vi "6221 Write.vi"(0 "Arbitrary Waveform\nArray of Channels":T1(array[cluster])=[[{"AC Frequency (kHz)"=0.0, " Initial AC Ampl. (p-p/2)"=0.0, "Final AC Ampl."=0.0, "Initial DC Value"=7.0, "Final DC Value"=1.0, "Constant/Tau"=2.0, "Gamma AC"=1.0, "String"="Channel 0 A", "Gamma DC/Beta"=1.0}, {"AC Frequency (kHz)"=40.0, " Initial AC Ampl. (p-p/2)"=0.0, "Final AC Ampl."=0.0, "Initial DC Value"=1.0, "Final DC Value"=1.0, "Constant/Tau"=2.0, "Gamma AC"=1.0, "String"="Channel 0 B", "Gamma DC/Beta"=1.0}, {"AC Frequency (kHz)"=40.0, " Initial AC Ampl. (p-p/2)"=0.0, "Final AC Ampl."=0.0, "Initial DC Value"=1.0, "Final DC Value"=1.0, "Constant/Tau"=2.0, "Gamma AC"=1.0, "String"="Channel 0 C", "Gamma DC/Beta"=1.0}, {"AC Frequency (kHz)"=0.0, " Initial AC Ampl. (p-p/2)"=0.0, "Final AC Ampl."=0.0, "Initial DC Value"=1.0, "Final DC Value"=7.0, "Constant/Tau"=2.0, "Gamma AC"=0.0, "String"="Channel 0 D", "Gamma DC/Beta"=1.0}, {"AC Frequency (kHz)"=0.0, " Initial AC Ampl. (p-p/2)"=0.0, "Final AC Ampl."=0.0, "Initial DC Value"=7.0, "Final DC Value"=6.0, "Constant/Tau"=2.0, "Gamma AC"=0.0, "String"="Channel 0 E", "Gamma DC/Beta"=1.0}], [{"AC Frequency (kHz)"=10.0, " Initial AC Ampl. (p-p/2)"=5.0, "Final AC Ampl."=0.0, "Initial DC Value"=0.2, "Final DC Value"=0.16, "Constant/Tau"=0.25, "Gamma AC"=1.0, "String"="Channel 1 A", "Gamma DC/Beta"=1.0}, {"AC Frequency (kHz)"=10.0, " Initial AC Ampl. (p-p/2)"=5.0, "Final AC Ampl."=0.0, "Initial DC Value"=0.16, "Final DC Value"=0.16, "Constant/Tau"=0.25, "Gamma AC"=1.0, "String"="Channel 1 B", "Gamma DC/Beta"=1.0}, {"AC Frequency (kHz)"=10.0, " Initial AC Ampl. (p-p/2)"=0.0, "Final AC Ampl."=0.0, "Initial DC Value"=0.0, "Final DC Value"=0.0, "Constant/Tau"=0.25, "Gamma AC"=1.0, "String"="Channel 1 C", "Gamma DC/Beta"=1.0}, {"AC Frequency (kHz)"=0.0, " Initial AC Ampl. (p-p/2)"=0.0, "Final AC Ampl."=0.0, "Initial DC Value"=1.0, "Final DC Value"=1.0, "Constant/Tau"=199.2, "Gamma AC"=0.0, "String"="Channel 1 D", "Gamma DC/Beta"=1.0}, {"AC Frequency (kHz)"=0.0, " Initial AC Ampl. (p-p/2)"=0.0, "Final AC Ampl."=0.0, "Initial DC Value"=1.0, "Final DC Value"=1.0, "Constant/Tau"=199.2, "Gamma AC"=0.0, "String"="Channel 1 E", "Gamma DC/Beta"=1.0}], [{"AC Frequency (kHz)"=10.0, " Initial AC Ampl. (p-p/2)"=0.0, "Final AC Ampl."=0.0, "Initial DC Value"=0.007, "Final DC Value"=0.06, "Constant/Tau"=0.0, "Gamma AC"=1.0, "String"="Channel 2 A", "Gamma DC/Beta"=1.0}, {"AC Frequency (kHz)"=10.0, " Initial AC Ampl. (p-p/2)"=0.0, "Final AC Ampl."=0.0, "Initial DC Value"=0.06, "Final DC Value"=0.06, "Constant/Tau"=0.0, "Gamma AC"=1.0, "String"="Channel 2 B", "Gamma DC/Beta"=1.0}, {"AC Frequency (kHz)"=10.0, " Initial AC Ampl. (p-p/2)"=0.0, "Final AC Ampl."=0.0, "Initial DC Value"=0.0, "Final DC Value"=0.0, "Constant/Tau"=0.0, "Gamma AC"=1.0, "String"="Channel 2 C", "Gamma DC/Beta"=1.0}, {"AC Frequency (kHz)"=0.0, " Initial AC Ampl. (p-p/2)"=0.0, "Final AC Ampl."=0.0, "Initial DC Value"=1.0, "Final DC Value"=1.0, "Constant/Tau"=199.2, "Gamma AC"=0.0, "String"="", "Gamma DC/Beta"=1.0}, {"AC Frequency (kHz)"=0.0, " Initial AC Ampl. (p-p/2)"=0.0, "Final AC Ampl."=0.0, "Initial DC Value"=1.0, "Final DC Value"=1.0, "Constant/Tau"=199.2, "Gamma AC"=0.0, "String"="", "Gamma DC/Beta"=1.0}], [{"AC Frequency (kHz)"=10.0, " Initial AC Ampl. (p-p/2)"=0.0, "Final AC Ampl."=0.0, "Initial DC Value"=1.0, "Final DC Value"=1.0, "Constant/Tau"=199.2, "Gamma AC"=1.0, "String"="Channel 3 A", "Gamma DC/Beta"=1.0}, {"AC Frequency (kHz)"=10.0, " Initial AC Ampl. (p-p/2)"=0.0, "Final AC Ampl."=0.0, "Initial DC Value"=1.0, "Final DC Value"=1.0, "Constant/Tau"=199.2, "Gamma AC"=1.0, "String"="Channel 3 B", "Gamma DC/Beta"=1.0}, {"AC Frequency (kHz)"=10.0, " Initial AC Ampl. (p-p/2)"=0.0, "Final AC Ampl."=0.0, "Initial DC Value"=1.0, "Final DC Value"=1.0, "Constant/Tau"=199.2, "Gamma AC"=1.0, "String"="Channel 3 C", "Gamma DC/Beta"=1.0}, {"AC Frequency (kHz)"=0.0, " Initial AC Ampl. (p-p/2)"=0.0, "Final AC Ampl."=0.0, "Initial DC Value"=1.0, "Final DC Value"=1.0, "Constant/Tau"=199.2, "Gamma AC"=0.0, "String"="", "Gamma DC/Beta"=1.0}, {"AC Frequency (kHz)"=0.0, " Initial AC Ampl. (p-p/2)"=0.0, "Final AC Ampl."=0.0, "Initial DC Value"=1.0, "Final DC Value"=1.0, "Constant/Tau"=199.2, "Gamma AC"=0.0, "String"="", "Gamma DC/Beta"=1.0}], [{"AC Frequency (kHz)"=10.0, " Initial AC Ampl. (p-p/2)"=0.0, "Final AC Ampl."=0.0, "Initial DC Value"=-0.1, "Final DC Value"=-0.04, "Constant/Tau"=199.2, "Gamma AC"=1.0, "String"="Channel 4 A", "Gamma DC/Beta"=1.0}, {"AC Frequency (kHz)"=10.0, " Initial AC Ampl. (p-p/2)"=0.0, "Final AC Ampl."=0.0, "Initial DC Value"=-0.1, "Final DC Value"=-0.04, "Constant/Tau"=199.2, "Gamma AC"=1.0, "String"="Channel 4 B", "Gamma DC/Beta"=1.0}, {"AC Frequency (kHz)"=10.0, " Initial AC Ampl. (p-p/2)"=0.0, "Final AC Ampl."=0.0, "Initial DC Value"=-0.1, "Final DC Value"=-0.04, "Constant/Tau"=199.2, "Gamma AC"=1.0, "String"="Channel 4 C", "Gamma DC/Beta"=1.0}, {"AC Frequency (kHz)"=0.0, " Initial AC Ampl. (p-p/2)"=0.0, "Final AC Ampl."=0.0, "Initial DC Value"=1.0, "Final DC Value"=1.0, "Constant/Tau"=199.2, "Gamma AC"=0.0, "String"="", "Gamma DC/Beta"=1.0}, {"AC Frequency (kHz)"=0.0, " Initial AC Ampl. (p-p/2)"=0.0, "Final AC Ampl."=0.0, "Initial DC Value"=1.0, "Final DC Value"=1.0, "Constant/Tau"=199.2, "Gamma AC"=0.0, "String"="", "Gamma DC/Beta"=1.0}], [{"AC Frequency (kHz)"=10.0, " Initial AC Ampl. (p-p/2)"=0.0, "Final AC Ampl."=0.0, "Initial DC Value"=-0.1, "Final DC Value"=-0.04, "Constant/Tau"=199.2, "Gamma AC"=1.0, "String"="Channel 5 A", "Gamma DC/Beta"=1.0}, {"AC Frequency (kHz)"=10.0, " Initial AC Ampl. (p-p/2)"=0.0, "Final AC Ampl."=0.0, "Initial DC Value"=-0.1, "Final DC Value"=-0.04, "Constant/Tau"=199.2, "Gamma AC"=1.0, "String"="Channel 5 B", "Gamma DC/Beta"=1.0}, {"AC Frequency (kHz)"=10.0, " Initial AC Ampl. (p-p/2)"=0.0, "Final AC Ampl."=0.0, "Initial DC Value"=-0.1, "Final DC Value"=-0.04, "Constant/Tau"=199.2, "Gamma AC"=1.0, "String"="Channel 5 C", "Gamma DC/Beta"=1.0}, {"AC Frequency (kHz)"=0.0, " Initial AC Ampl. (p-p/2)"=0.0, "Final AC Ampl."=0.0, "Initial DC Value"=1.0, "Final DC Value"=1.0, "Constant/Tau"=199.2, "Gamma AC"=0.0, "String"="", "Gamma DC/Beta"=1.0}, {"AC Frequency (kHz)"=0.0, " Initial AC Ampl. (p-p/2)"=0.0, "Final AC Ampl."=0.0, "Initial DC Value"=1.0, "Final DC Value"=1.0, "Constant/Tau"=199.2, "Gamma AC"=0.0, "String"="", "Gamma DC/Beta"=1.0}], [{"AC Frequency (kHz)"=10.0, " Initial AC Ampl. (p-p/2)"=0.0, "Final AC Ampl."=0.0, "Initial DC Value"=-0.1, "Final DC Value"=-0.04, "Constant/Tau"=199.2, "Gamma AC"=1.0, "String"="Channel 6 A", "Gamma DC/Beta"=1.0}, {"AC Frequency (kHz)"=10.0, " Initial AC Ampl. (p-p/2)"=0.0, "Final AC Ampl."=0.0, "Initial DC Value"=-0.1, "Final DC Value"=-0.04, "Constant/Tau"=199.2, "Gamma AC"=1.0, "String"="Channel 6 B", "Gamma DC/Beta"=1.0}, {"AC Frequency (kHz)"=10.0, " Initial AC Ampl. (p-p/2)"=0.0, "Final AC Ampl."=0.0, "Initial DC Value"=-0.1, "Final DC Value"=-0.04, "Constant/Tau"=199.2, "Gamma AC"=1.0, "String"="Channel 6 C", "Gamma DC/Beta"=1.0}, {"AC Frequency (kHz)"=0.0, " Initial AC Ampl. (p-p/2)"=0.0, "Final AC Ampl."=0.0, "Initial DC Value"=1.0, "Final DC Value"=1.0, "Constant/Tau"=199.2, "Gamma AC"=0.0, "String"="", "Gamma DC/Beta"=1.0}, {"AC Frequency (kHz)"=0.0, " Initial AC Ampl. (p-p/2)"=0.0, "Final AC Ampl."=0.0, "Initial DC Value"=1.0, "Final DC Value"=1.0, "Constant/Tau"=199.2, "Gamma AC"=0.0, "String"="", "Gamma DC/Beta"=1.0}], [{"AC Frequency (kHz)"=10.0, " Initial AC Ampl. (p-p/2)"=0.0, "Final AC Ampl."=0.0, "Initial DC Value"=-0.1, "Final DC Value"=-0.04, "Constant/Tau"=199.2, "Gamma AC"=1.0, "String"="Channel 7 A", "Gamma DC/Beta"=1.0}, {"AC Frequency (kHz)"=10.0, " Initial AC Ampl. (p-p/2)"=0.0, "Final AC Ampl."=0.0, "Initial DC Value"=-0.1, "Final DC Value"=-0.04, "Constant/Tau"=199.2, "Gamma AC"=1.0, "String"="Channel 7 B", "Gamma DC/Beta"=1.0}, {"AC Frequency (kHz)"=10.0, " Initial AC Ampl. (p-p/2)"=0.0, "Final AC Ampl."=0.0, "Initial DC Value"=-0.1, "Final DC Value"=-0.04, "Constant/Tau"=199.2, "Gamma AC"=1.0, "String"="Channel 7 C", "Gamma DC/Beta"=1.0}, {"AC Frequency (kHz)"=0.0, " Initial AC Ampl. (p-p/2)"=0.0, "Final AC Ampl."=0.0, "Initial DC Value"=1.0, "Final DC Value"=1.0, "Constant/Tau"=199.2, "Gamma AC"=0.0, "String"="", "Gamma DC/Beta"=1.0}, {"AC Frequency (kHz)"=0.0, " Initial AC Ampl. (p-p/2)"=0.0, "Final AC Ampl."=0.0, "Initial DC Value"=1.0, "Final DC Value"=1.0, "Constant/Tau"=199.2, "Gamma AC"=0.0, "String"="", "Gamma DC/Beta"=1.0}]] {"Gamma DC/Beta" format="%.2f"; "Gamma AC" format="%.2f"; "Constant/Tau" min=0.0 max=240.0 format="%.4f"; "Final DC Value" format="%.3f"; "Initial DC Value" format="%.3f"; "Final AC Ampl." format="%.3f"; "Initial AC Ampl. (p-p/2)" format="%.3f"; "AC Frequency (kHz)" format="%.2f"}, 2 "Channel to plot":i32 min=0 max=7, 3 "Unit Conversions":u16[](array[ring])=[0, 0, 2, 3, 4, 0, 0, 0] items=["Volts-to-Volts Power Law", "Evaporation Formula", "Dimple Evaporation"], 4 "Interval Lengths (ms)":dbl[](array[numeric])=[120.0, 16.0, 484.0, 700.0, 100.0] format="%.3f", 5 "Channel Controls":bool[](array[boolean])=[TRUE, TRUE, FALSE, FALSE, FALSE, FALSE, FALSE, FALSE], 6 "ON or OFF?":bool[](array[boolean])=[TRUE, TRUE, TRUE, FALSE, FALSE], 11 "error in":errorcluster, 12 "Dither Control":u16(ring)=1 items=["Disable Dither", "Enable Dither"]) -> (9 "Sampling Rate":dbl=2882.3529411764707 format="%.2f", 10 "= Total Waveform\nTime (ms)":dbl=1420.0 format="%.3f", 13 "Waveform on Channel to Plot":cluster{dbl[], dbl[]}(graph), 14 "signal out":waveform(dbl)[](graph)=[{"t0"=timestamp(0 s since 1904-01-01), "dt"=0.00034693877551020405, "Y"=array[4091 elements]}, {"t0"=timestamp(0 s since 1904-01-01), "dt"=0.00034693877551020405, "Y"=array[4091 elements]}], 15 "error out":errorcluster)   [LabVIEW 2013]
uses:
  <vilib>/Utility/error.llb/DialogType.ctl
  <vilib>/DAQmx/write.llb/DAQmx Write (Analog 1D Wfm NChan NSamp).vi
  <vilib>/DAQmx/configure/timing.llb/DAQmx Timing (Sample Clock).vi
  <vilib>/DAQmx/create/channels.llb/DAQmx Create Channel (CO-Pulse Generation-Frequency).vi
  <vilib>/DAQmx/configure/timing.llb/DAQmx Timing (Implicit).vi
  <vilib>/DAQmx/configure/trigger.llb/DAQmx Start Trigger (Digital Edge).vi
  <vilib>/DAQmx/miscellaneous.llb/DAQmx Fill In Error Info.vi
  <resource>/objmgr/daqmx.rc
panel:
  in  "Case Constant\n(See Context Help) 3":bool=TRUE
  in  "Case Constant\n(See Context Help) 2":bool
  in  "Dither Control":u16
  in  "Case Constant\n(See Context Help)":bool
  in  "Dither Control":u16
  out "Pmod Graph":dbl[][](graph)
  out "wvfrm size":i32=4091
  out "x+y 2":dbl=1.42
  out "Numeric":i32=287
  out "6221 counter task out":refnum<k21>="Counter Output"
  out "6221 adiabatic loading task out":refnum<k21>="Adiabatic Loading"
  out "Array":dbl[][](array[numeric])
  out "6221 Status":string="PCI-6221 OK"
  out "total points":dbl=4092.0 format="%.2f"
  out "Points per Segment":dbl[](array[numeric])=[345.0, 46.0, 1395.0, 2017.0, 288.0] format="%.2f"
  # "Warning! Constant for interval A does not set all intervals for 86 Sr frequency"
  # "Controls"
  # "Volts to Volts Power Law Formula\nf100=DCinitial +(DCfinal-DCinitial)*(time/intervaltime)**gammaDC;"
  # "Don't change"
  # "Note: B-field to Voltage\nConversion not yet\nimplemented.  Must \ninsert appropriate\nformulae."
  # "CH 0"
  # "CH 1"
  # "Evaporation Formula\nf100=Initial/((1+(time/tau))**beta)+Final;"
  # "Initial DC = U1, Constant = Tau\nGamma DC = Beta"
  # "Interval A"
  # "Interval B"
  # "Interval C"
  # "Interval D"
  # "Interval E"
  # "Interval F"
  # "Output"
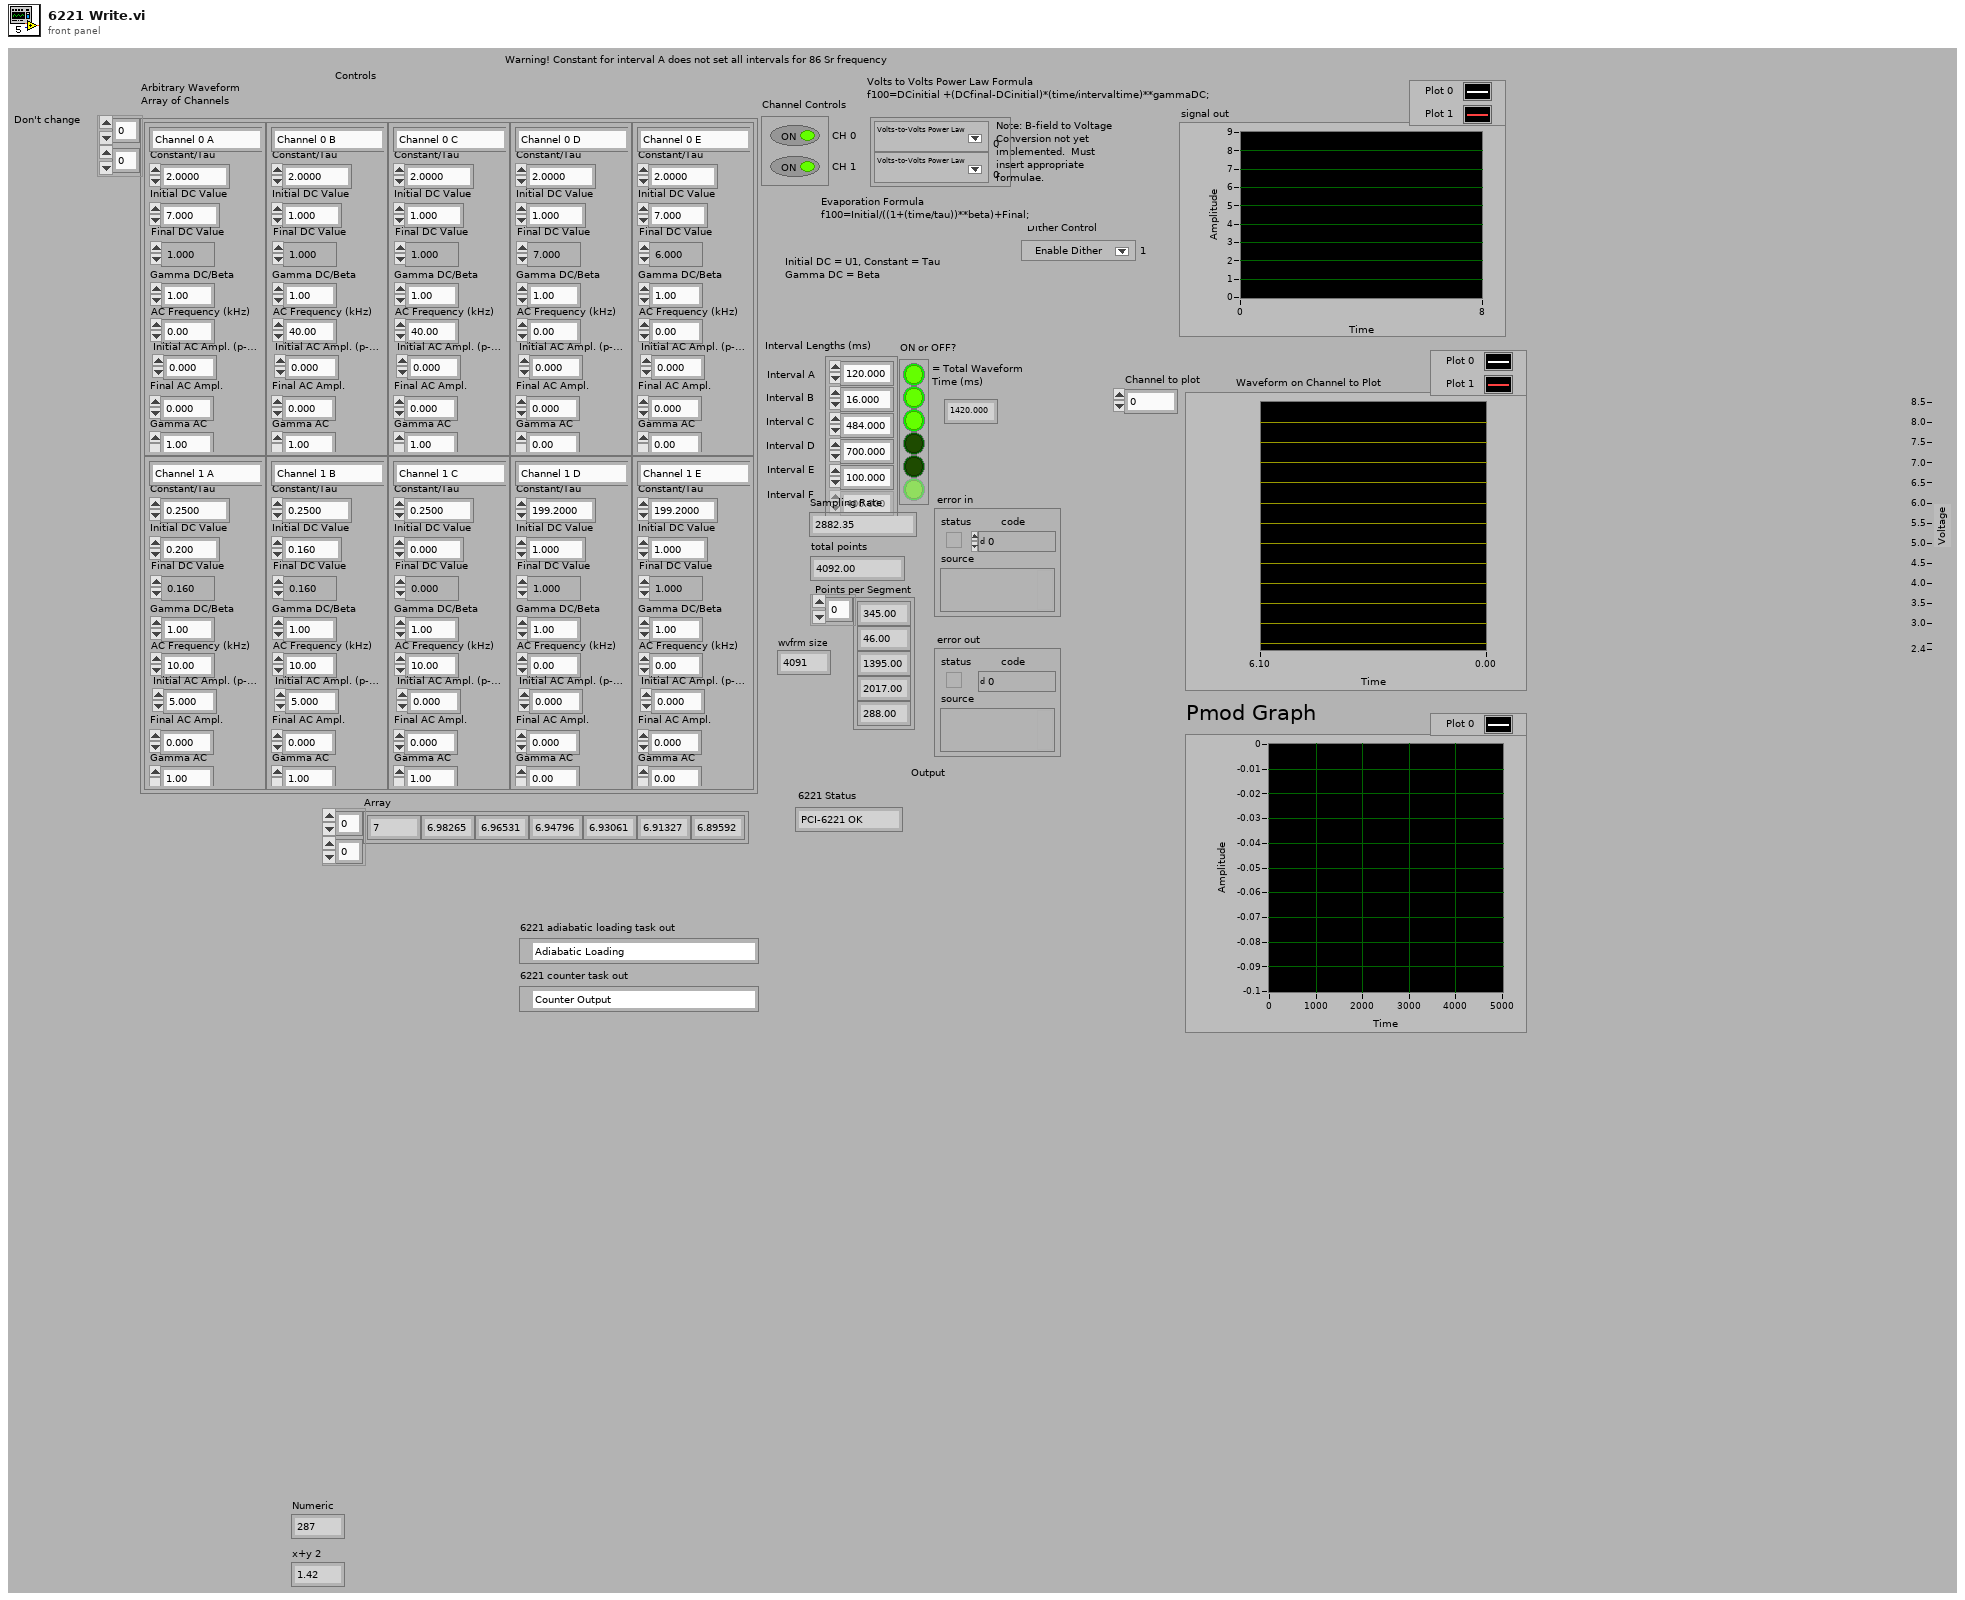
[diagram p1: front panel]
types:
  T1 = cluster{"AC Frequency (kHz)":dbl, " Initial AC Ampl. (p-p/2)":dbl, "Final AC Ampl.":dbl, "Initial DC Value":dbl, "Final DC Value":dbl, "Constant/Tau":dbl, "Gamma AC":dbl, "String":string, "Gamma DC/Beta":dbl}[][]
  T2 = cluster{"AC Frequency (kHz)":dbl, " Initial AC Ampl. (p-p/2)":dbl, "Final AC Ampl.":dbl, "Initial DC Value":dbl, "Final DC Value":dbl, "Constant/Tau":dbl, "Gamma AC":dbl, "String":string, "Gamma DC/Beta":dbl}
  T3 = typedef "DialogType.ctl" = u16
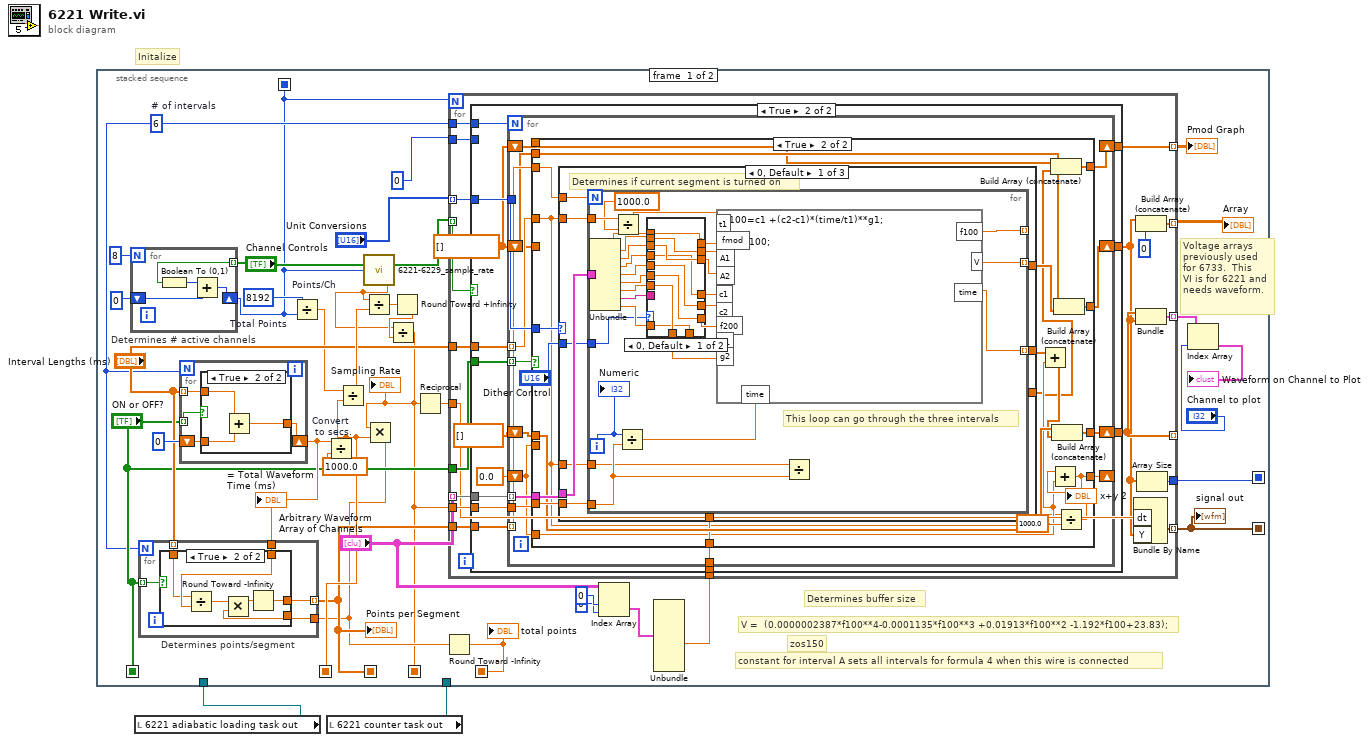
[diagram p0: block diagram]
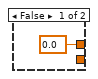
[diagram p2: hidden frame]
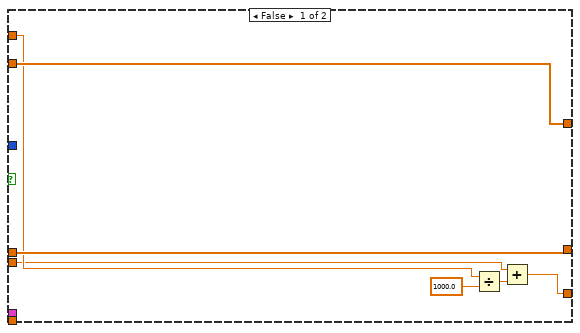
[diagram p5: hidden frame]
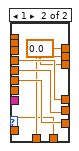
[diagram p6: hidden frame]
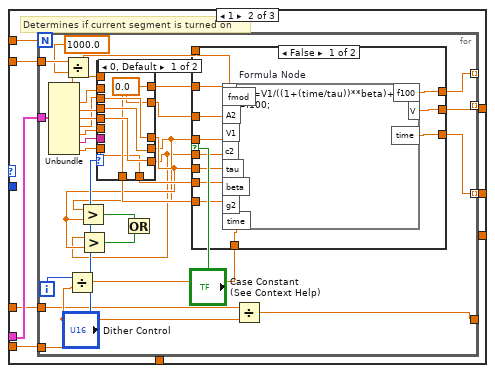
[diagram p7: hidden frame]
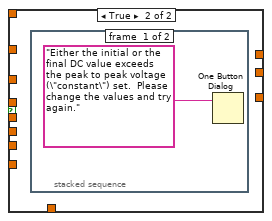
[diagram p8: hidden frame]
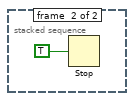
[diagram p9: hidden frame]
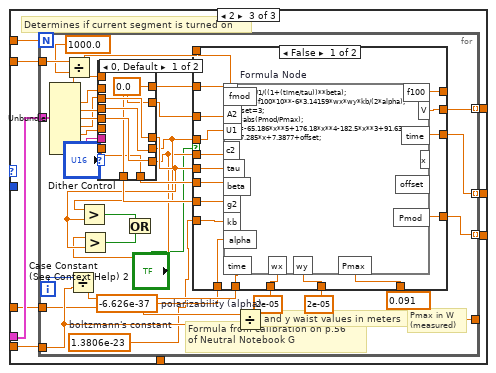
[diagram p11: hidden frame]
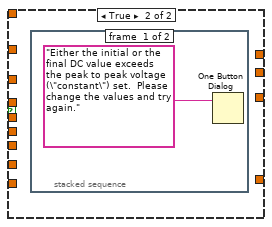
[diagram p12: hidden frame]
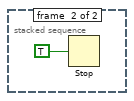
[diagram p13: hidden frame]
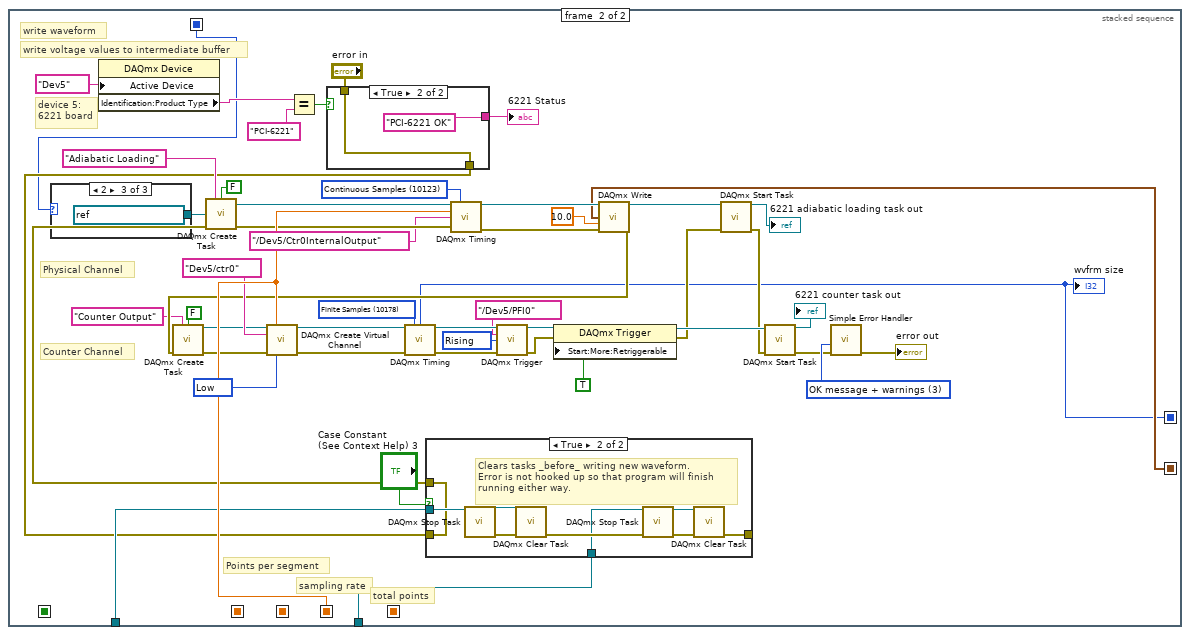
[diagram p15: hidden frame]
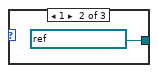
[diagram p17: hidden frame]
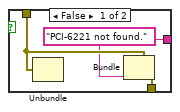
[diagram p19: hidden frame]
diagram:
  # "Initalize"
  n1 = local read "6221 adiabatic loading task out"() -> (w2:refnum<k21>)
  n2 = local read "6221 counter task out"() -> (w1:refnum<k21>)
  n3 = stacked-sequence {
    seq-local: [w10 _] -> [_ w356]
    seq-local: [w22 _] -> [_ _]
    seq-local: ["ON or OFF?" _] -> [_ _]
    seq-local: [w19 _] -> [_ _]
    seq-local: [w24 _] -> [_ _]
    seq-local: [w8 _] -> [_ w330]
    seq-local: [w3 _] -> [_ w331]
    seq-local: [w7 _] -> [_ w329]
    tunnel: w2 -> [_ w341]
    tunnel: w1 -> [_ w342]
    frame #0 {
      w6 = 6  # # of intervals
      w38 = 8192  # Total Points
      # "Voltage arrays\npreviously used\nfor 6733.  This\nVI is for 6221 and\nneeds waveform."
      # "zos150"
      # "Determines buffer size"
      # "constant for interval A sets all intervals for formula 4 when this wire is connected"
      # "V =  (0.0000002387*f100**4-0.0001135*f100**3 +0.01913*f100**2 -1.192*f100+23.83);"
      n4 = for "Determines # active channels" {
        N: 8 -> [_]
        tunnel: "Channel Controls" -> [w62] mode=indexing
        shift-right: [w59] -> w3
        shift-left: 0 -> [w60]
        n5 = Boolean To (0,1)(Boolean=w62) -> (0, 1=w61:i16)
        n6 = Add(x=w61, y=w60) -> (x+y=w59:i32)
      }
      n7 = for {
        N: w6 -> [_]
        tunnel: "Interval Lengths (ms)" -> [w52] mode=indexing
        tunnel: "ON or OFF?" -> [w54] mode=indexing
        shift-right: [w51] -> w25
        shift-left: 0 -> [w53]
        n8 = case shown="True" w54 {
          tunnel: w53 -> [w55 w58]
          tunnel: w52 -> [_ w57]
          tunnel: [w55 w56] -> w51
          frame False {
          }
          frame True {
            n9 = Add(x=w57, y=w58) -> (x+y=w56:dbl)
          }
        }
      }
      "= Total Waveform\nTime (ms)" <- w25
      n10 = Divide "Points/Ch"(x=w38, y=w3) -> (x/y=w23:dbl)
      n11 = Divide "Convert\n to secs."(x=w25, y=1000.0) -> (x/y=w24:dbl)
      n12 = Divide(x=w23, y=w24) -> (x/y=w30:dbl)
      n13 = call "6221-6229_sample_rate.vi"("# of output channels"=w3) -> ("Sampling rate"=w4:dbl)
      n14 = Divide(x=w4, y=w30) -> (x/y=w29:dbl)
      n15 = Round Toward +Infinity(x=w29) -> (ceil(x): smallest int >= x=w28:dbl)
      n16 = Divide(x=w4, y=w28) -> (x/y=w10:dbl)
      "Sampling Rate" <- w10
      n17 = Multiply(x=w10, y=w24) -> (x*y=w20:dbl)
      n18 = for "Determines points/segment" {
        N: w6 -> [_]
        tunnel: "ON or OFF?" -> [w43] mode=indexing
        tunnel: "Interval Lengths (ms)" -> [w42] mode=indexing
        tunnel: w25 -> [w41]
        tunnel: [w40] -> w22 mode=indexing
        tunnel: w20 -> [w39]
        n19 = case shown="True" w43 {
          tunnel: w42 -> [_ w49]
          tunnel: w41 -> [_ w50]
          tunnel: [0.0 w46] -> w40
          tunnel: w39 -> [_ w47]
          frame False {
          }
          frame True {
            n20 = Divide(x=w49, y=w50) -> (x/y=w48:dbl)
            n21 = Multiply(x=w48, y=w47) -> (x*y=w45:dbl)
            n22 = Round Toward -Infinity(1:w45) -> (0:w46:dbl)
          }
        }
      }
      "Points per Segment" <- w22
      n23 = Reciprocal(x=w10) -> (1/x=w9:dbl)
      n24 = Round Toward -Infinity(1:w20) -> (0:w19:dbl)
      "total points" <- w19
      n25 = Index Array(array="Arbitrary Waveform\nArray of Channels", index (row)=0, index (col)=0 ("disabled index (col)")) -> (element=w14:T2)
      n26 = Unbundle(w14) -> ("Constant/Tau"=w13:dbl)  [unwired: 8 out]
      n27 = for {
        N: w3 -> [_]
        tunnel: "Channel Controls" -> [w81] mode=indexing
        tunnel: 0 -> [w80]
        tunnel: "Unit Conversions" -> [w78] mode=indexing
        tunnel: "Arbitrary Waveform\nArray of Channels" -> [w79] mode=indexing
        tunnel: w22 -> [w77]
        tunnel: w10 -> [w76]
        tunnel: "Interval Lengths (ms)" -> [w75]
        tunnel: "ON or OFF?" -> [w74]
        tunnel: [w67] -> _ mode=indexing
        tunnel: [w71] -> w18 mode=indexing
        tunnel: [w73] -> w26 mode=indexing
        tunnel: w13 -> [w70]
        tunnel: w9 -> [w69]
        tunnel: [w68] -> w8 mode=indexing
        tunnel: [w65] -> w7
        tunnel: w6 -> [w64]
        tunnel: [w63] -> w5 mode=indexing
        n28 = case shown="True" w81 {
          tunnel: w80 -> [_ _]
          tunnel: w79 -> [_ w95]
          tunnel: w78 -> [_ w94]
          tunnel: w77 -> [_ w93]
          tunnel: w76 -> [_ w92]
          tunnel: w75 -> [_ w91]
          tunnel: w74 -> [_ w90]
          tunnel: [_ w89] -> w66
          tunnel: w70 -> [_ w88]
          tunnel: [_ w86] -> w67
          tunnel: w64 -> [_ w84]
          tunnel: [_ w82] -> w63
          frame False {
          }
          frame True {
            w83 = dbl[] []
            n29 = for {
              N: w84 -> [_]
              tunnel: w95 -> [w108] mode=indexing
              tunnel: w94 -> [w110]
              tunnel: w93 -> [w109] mode=indexing
              tunnel: w92 -> [w107]
              tunnel: w91 -> [w106] mode=indexing
              tunnel: w90 -> [w105] mode=indexing
              shift-right: [w99] -> w86
              shift-left: dbl[] [] -> [w104]
              shift-right: [w103] -> _
              shift-left: 0.0 -> [w98]
              shift-right: [w102] -> w89
              shift-left: w83 -> [w101]
              tunnel: w88 -> [w100]
              shift-right: [w96] -> w82
              shift-left: w83 -> [w97]
              n30 = case shown="True" w105 {
                tunnel: w110 -> [_ w131]
                tunnel: w109 -> [_ w127]
                tunnel: w108 -> [_ w138]
                tunnel: w107 -> [_ w137]
                tunnel: w106 -> [w113 w121]
                tunnel: [w117 w136] -> w99
                tunnel: w104 -> [w117 w135]
                tunnel: [w112 w128] -> w103
                tunnel: [w116 w134] -> w102
                tunnel: w101 -> [_ w132]
                tunnel: w101 -> [w116 _]
                tunnel: w100 -> [_ w129]
                tunnel: w98 -> [_ w122]
                tunnel: w98 -> [w111 _]
                tunnel: [_ w119] -> w96
                tunnel: w97 -> [_ w118]
                frame False {
                  n31 = Divide(x=w113, y=1000.0) -> (x/y=w115:dbl)
                  n32 = Add(x=w111, y=w115) -> (x+y=w112:dbl)
                }
                frame True {
                  n33 = case shown="0, Default" w131 {
                    tunnel: w127 -> [w146 w195 w260]
                    tunnel: w138 -> [w145 w194 w259]
                    tunnel: w137 -> [w141 w190 w255]
                    tunnel: w121 -> [w144 w193 w258]
                    tunnel: [w143 w192 w257] -> w133
                    tunnel: [w142 w191 w256] -> w124
                    tunnel: w121 -> [w140 w189 w254]
                    tunnel: "Dither Control" -> [w139 _ _]
                    tunnel: w129 -> [_ _ _]
                    tunnel: [_ _ w253] -> w120
                    frame 0, Default {
                      # "Determines if current segment is turned on"
                      n34 = for {
                        N: w146 -> [_]
                        tunnel: w145 -> [w175]
                        tunnel: w141 -> [w154]
                        tunnel: w144 -> [w174]
                        tunnel: [w152] -> w143 mode=indexing
                        tunnel: [w153] -> w142 mode=indexing
                        tunnel: [w151] -> _ mode=indexing
                        tunnel: w140 -> [w149]
                        tunnel: w139 -> [w150]
                        i -> [w172]
                        # "Volts-to-Volts Power Law"
                        # "This loop can go through the three intervals"
                        n35 = Unbundle(w175) -> ("AC Frequency (kHz)"=w168:dbl, "Initial AC Ampl. (p-p/2)"=w167:dbl, "Final AC Ampl."=w166:dbl, "Initial DC Value"=w147:dbl, "Final DC Value"=w165:dbl, "Constant/Tau"=w169:dbl, "Gamma AC"=w170:dbl, "String"=w171:string, "Gamma DC/Beta"=w156:dbl)
                        n36 = Divide(x=w174, y=1000.0) -> (x/y=w164:dbl)
                        n37 = Divide(x=w172, y=w154) -> (x/y=w148:dbl)
                        n38 = case shown="0, Default" w150 {
                          tunnel: w171 -> [_ _]
                          tunnel: w170 -> [w177 _]
                          tunnel: w169 -> [w178 w186]
                          tunnel: w168 -> [w183 _]
                          tunnel: w167 -> [w182 _]
                          tunnel: w166 -> [w181 _]
                          tunnel: w147 -> [w180 w188]
                          tunnel: w165 -> [w179 w187]
                          tunnel: [w183 w185] -> w163
                          tunnel: [w182 w185] -> w162
                          tunnel: [w181 w185] -> w161
                          tunnel: [w180 w188] -> w160
                          tunnel: [w179 w187] -> w159
                          tunnel: [w178 w186] -> w158
                          tunnel: [w177 w185] -> w157
                          tunnel: w156 -> [w176 w184]
                          tunnel: [w176 w184] -> w155
                          frame 0, Default {
                          }
                          frame 1 {
                            w185 = 0.0 ("AC Frequency (kHz)")
                          }
                        }
                        n39 = formula code="f100=c1 +(c2-c1)*(time/t1)**g1;\n\nV = f100;"("c1"=w160, "time"=w148, "t1"=w164, "c2"=w159, "f200"=w158, "fmod"=w163, "A1"=w162, "A2"=w161, "g1"=w155, "g2"=w157) -> ("f100"=w151:dbl, "time"=w153:dbl, "V"=w152:dbl)
                        n40 = Divide(x=w149, y=w154) -> ()  [unwired: 1 out]
                        "Numeric" <- w172
                      }
                    }
                    frame 1 {
                      # "Determines if current segment is turned on"
                      n41 = for {
                        N: w195 -> [_]
                        tunnel: w194 -> [w226]
                        tunnel: w190 -> [w210]
                        tunnel: w193 -> [w222]
                        tunnel: [w225] -> w192 mode=indexing
                        tunnel: [w224] -> w191 mode=indexing
                        tunnel: [w223] -> _ mode=indexing
                        tunnel: [w209] -> _
                        tunnel: w189 -> [w197]
                        i -> [w220]
                        n42 = Unbundle(w226) -> ("AC Frequency (kHz)"=w203:dbl, "Final AC Ampl."=w204:dbl, "Initial DC Value"=w207:dbl, "Final DC Value"=w206:dbl, "Constant/Tau"=w205:dbl, "Gamma AC"=w218:dbl, "String"=w219:string, "Gamma DC/Beta"=w213:dbl)  [unwired: 1 out]
                        n43 = Divide(x=w222, y=1000.0) -> (x/y=w217:dbl)
                        n44 = Divide(x=w220, y=w210) -> (x/y=w211:dbl)
                        n45 = case shown="0, Default" "Dither Control" {
                          tunnel: w219 -> [_ _]
                          tunnel: w218 -> [_ w248]
                          tunnel: w206 -> [w243 w249]
                          tunnel: w204 -> [_ w252]
                          tunnel: w205 -> [w245 w251]
                          tunnel: w207 -> [w244 w250]
                          tunnel: [w242 w246] -> w216
                          tunnel: [w242 w252] -> w215
                          tunnel: [w245 w251] -> w200
                          tunnel: [w244 w250] -> w199
                          tunnel: [w243 w249] -> w198
                          tunnel: [w242 w248] -> w214
                          tunnel: w213 -> [w241 w247]
                          tunnel: [w241 w247] -> w212
                          tunnel: w203 -> [_ w246]
                          frame 0, Default {
                            w242 = 0.0 ("AC Frequency (kHz)")
                          }
                          frame 1 {
                          }
                        }
                        n46 = Greater?(x=w199, y=w200) -> (0:w201:bool)
                        n47 = Greater?(x=w198, y=w200) -> (0:w202:bool)
                        n48 = Or(x=w201, y=w202) -> ()  [unwired: 1 out]
                        n49 = case shown="False" "Case Constant\n(See Context Help)" {
                          tunnel: [w238 _] -> w225
                          tunnel: [w237 _] -> w224
                          tunnel: [w236 _] -> w223
                          tunnel: w217 -> [w235 _]
                          tunnel: w216 -> [w234 _]
                          tunnel: w215 -> [w233 _]
                          tunnel: w214 -> [w232 _]
                          tunnel: w212 -> [w231 _]
                          tunnel: w211 -> [w230 _]
                          tunnel: w199 -> [w229 _]
                          tunnel: w198 -> [w228 _]
                          tunnel: w200 -> [w227 _]
                          frame False {
                            # "Evaporative Cooling"
                            n50 = formula code="f100=V1/((1+(time/tau))**beta)+c2;\nV=f100;"("V1"=w229, "time"=w230, "t1"=w235, "c2"=w228, "tau"=w227, "fmod"=w234, "A2"=w233, "beta"=w231, "g2"=w232) -> ("f100"=w236:dbl, "time"=w237:dbl, "V"=w238:dbl)
                          }
                          frame True {
                            n51 = stacked-sequence {
                              frame #0 {
                                n52 = One Button Dialog(message="Either the initial or the final DC value exceeds the peak to peak voltage (\"constant\") set.  Please change the values and try again.") -> ()  [unwired: 1 in, 1 out]
                              }
                              frame #1 {
                                n53 = Stop(stop? (T)=TRUE) -> ()
                              }
                            }
                          }
                        }
                        n54 = Divide(x=w197, y=w210) -> (x/y=w209:dbl)
                      }
                    }
                    frame 2 {
                      # "Determines if current segment is turned on"
                      n55 = for {
                        N: w260 -> [_]
                        tunnel: w259 -> [w296]
                        tunnel: w255 -> [w281]
                        tunnel: w258 -> [w293]
                        tunnel: [w295] -> w257 mode=indexing
                        tunnel: [w294] -> w256 mode=indexing
                        tunnel: [w280] -> _
                        tunnel: w254 -> [w268]
                        tunnel: [w261] -> w253 mode=indexing
                        i -> [w291]
                        w266 = -6.626e-37  # polarizability (alpha)
                        w265 = 1.3806e-23  # boltzmann's constant
                        # "Pmax in W\n(measured)"
                        # "x and y waist values in meters"
                        # "Formula from calibration on p.56 \nof Neutral Notebook G"
                        n56 = Unbundle(w296) -> ("AC Frequency (kHz)"=w274:dbl, "Final AC Ampl."=w275:dbl, "Initial DC Value"=w278:dbl, "Final DC Value"=w277:dbl, "Constant/Tau"=w276:dbl, "Gamma AC"=w289:dbl, "String"=w290:string, "Gamma DC/Beta"=w284:dbl)  [unwired: 1 out]
                        n57 = Divide(x=w293, y=1000.0) -> (x/y=w288:dbl)
                        n58 = Divide(x=w291, y=w281) -> (x/y=w282:dbl)
                        n59 = case shown="0, Default" "Dither Control" {
                          tunnel: w290 -> [_ _]
                          tunnel: w289 -> [_ w324]
                          tunnel: w277 -> [w319 w325]
                          tunnel: w275 -> [_ w328]
                          tunnel: w276 -> [w321 w327]
                          tunnel: w278 -> [w320 w326]
                          tunnel: [w318 w322] -> w287
                          tunnel: [w318 w328] -> w286
                          tunnel: [w321 w327] -> w271
                          tunnel: [w320 w326] -> w270
                          tunnel: [w319 w325] -> w269
                          tunnel: [w318 w324] -> w285
                          tunnel: w284 -> [w317 w323]
                          tunnel: [w317 w323] -> w283
                          tunnel: w274 -> [_ w322]
                          frame 0, Default {
                            w318 = 0.0 ("AC Frequency (kHz)")
                          }
                          frame 1 {
                          }
                        }
                        n60 = Greater?(x=w270, y=w271) -> (0:w272:bool)
                        n61 = Greater?(x=w269, y=w271) -> (0:w273:bool)
                        n62 = Or(x=w272, y=w273) -> ()  [unwired: 1 out]
                        n63 = case shown="False" "Case Constant\n(See Context Help) 2" {
                          tunnel: [w314 _] -> w295
                          tunnel: [w313 _] -> w294
                          tunnel: [w312 _] -> _
                          tunnel: w288 -> [w311 _]
                          tunnel: w287 -> [w310 _]
                          tunnel: w286 -> [w309 _]
                          tunnel: w285 -> [w308 _]
                          tunnel: w283 -> [w307 _]
                          tunnel: w282 -> [w306 _]
                          tunnel: w270 -> [w299 _]
                          tunnel: w269 -> [w305 _]
                          tunnel: w271 -> [w304 _]
                          tunnel: w266 -> [w303 _]
                          tunnel: w265 -> [w302 _]
                          tunnel: 2e-05 -> [w301 _]
                          tunnel: 2e-05 -> [w300 _]
                          tunnel: 0.091 -> [w298 _]
                          tunnel: [w297 _] -> w261
                          frame False {
                            # "Evaporative Cooling"
                            n64 = formula code="f100=U1/((1+(time/tau))**beta);\nPmod=f100*10**-6*3.14159*wx*wy*kb/(2*alpha);\noffset=3;\nx=abs(Pmod/Pmax);\nV=-65.186*x**5+176.18*x**4-182.5*x**3+91.63*x**2-27.285*x+7.3877+offset;"("U1"=w299, "time"=w306, "t1"=w311, "c2"=w305, "tau"=w304, "fmod"=w310, "A2"=w309, "beta"=w307, "g2"=w308, "kb"=w302, "alpha"=w303, "wx"=w300, "wy"=w301, "Pmax"=w298) -> ("f100"=w312:dbl, "time"=w313:dbl, "V"=w314:dbl, "Pmod"=w297:dbl)  [unwired: 2 out]
                          }
                          frame True {
                            n65 = stacked-sequence {
                              frame #0 {
                                n66 = One Button Dialog(message="Either the initial or the final DC value exceeds the peak to peak voltage (\"constant\") set.  Please change the values and try again.") -> ()  [unwired: 1 in, 1 out]
                              }
                              frame #1 {
                                n67 = Stop(stop? (T)=TRUE) -> ()
                              }
                            }
                          }
                        }
                        n68 = Divide(x=w268, y=w281) -> (x/y=w280:dbl)
                      }
                    }
                  }
                  n69 = Add(x=w124, y=w122) -> (x+y=w123:dbl[])
                  n70 = Build Array (concatenate)(w118, w120) -> (w119:dbl[])
                  n71 = Build Array (concatenate)(w135, w123) -> (w136:dbl[])
                  n72 = Build Array (concatenate)(w132, w133) -> (w134:dbl[])
                  n73 = Divide(x=w121, y=1000.0) -> (x/y=w126:dbl)
                  n74 = Add(x=w126, y=w122) -> (x+y=w128:dbl)
                  "x+y 2" <- w128
                }
              }
            }
          }
        }
        n75 = Bundle By Name("dt"=w69, "Y"=w66) -> (w68:waveform(dbl))  [unwired: 1 in]
        n76 = Build Array (concatenate)(w66, 0) -> (w71:dbl[])
        n77 = Bundle(w67, w66) -> (w73:cluster{dbl[], dbl[]})  [unwired: 1 in]
        n78 = Array Size(array=w66) -> (size(s)=w65:i32)
      }
      "signal out" <- w8
      "Array" <- w18
      "Pmod Graph" <- w5
      n79 = Index Array(array=w26, index="Channel to plot") -> (element=→"Waveform on Channel to Plot":cluster{dbl[], dbl[]})
    }
    frame #1 {
      w363 = 10214 items=["High"=10192, "Low"=10214] ("idle state")
      w365 = 10280 items=["Rising"=10280, "Falling"=10171] ("edge")
      w371 = 10178 items=["Finite Samples"=10178, "Continuous Samples"=10123, "Hardware Timed Single Point"=12522] ("sample mode")
      w374 = T3 3 items=["no dialog", "OK message", "continue or stop message", "OK message + warnings", "continue/stop + warnings"] ("type of dialog (OK msg:1)")
      w375 = 10123 items=["Finite Samples"=10178, "Continuous Samples"=10123, "Hardware Timed Single Point"=12522] ("sample mode")
      # "Physical Channel"
      # "Counter Channel"
      # "sampling rate"
      # "total points"
      # "Points per segment"
      # "write voltage values to intermediate buffer"
      # "write waveform"
      # "device 5:\n6221 board"
      n80 = case shown="2" w331 {
        tunnel: [_ refnum<k21> "NI6221 A0 00" ("global virtual channels") refnum<k21> "NI6221 A0 00:01" ("global virtual channels")] -> w332
        frame 0, Default {
          # "Program no channels"
        }
        frame 1 {
        }
        frame 2 {
        }
      }
      n81 = property class="DAQmx Device"("Active Device"=tag "Dev5") -> ("Identification:Product Type"=w336:string)  [unwired: 2 in, 2 out]
      n82 = Equal?(x=w336, y="PCI-6221") -> (x = y?=w378:bool)
      n83 = case shown="True" w378 {
        tunnel: [w393 "PCI-6221 OK"] -> w377
        tunnel: "error in" -> [w394 w395]
        tunnel: [w392 w395] -> w339
        frame False {
          w393 = "PCI-6221 not found."
          n84 = Unbundle(w394) -> ()  [unwired: 3 out]
          n85 = Bundle(cluster=w394, "source"=w393) -> (w392:errorcluster)  [unwired: 2 in]
        }
        frame True {
        }
      }
      "6221 Status" <- w377
      n86 = case shown="True" "Case Constant\n(See Context Help) 3" {
        tunnel: w342 -> [_ w386]
        tunnel: w341 -> [_ w385]
        tunnel: w339 -> [w382 w384]
        tunnel: [w382 w384] -> w338
        tunnel: [_ w383] -> _
        frame False {
        }
        frame True {
          # "Clears tasks _before_ writing new waveform.\nError is not hooked up so that program will finish\nrunning either way."
          n87 = call <vilib>:"DAQmx Stop Task.vi"("task/channels in"=w385) -> ("task out"=w390:refnum<k21>, "error out"=w391:errorcluster)  [unwired: 13 in]
          n88 = call <vilib>:"DAQmx Clear Task.vi"("task in"=w390, "error in"=w391) -> ("error out"=w387:errorcluster)  [unwired: 13 in]
          n89 = call <vilib>:"DAQmx Stop Task.vi"("task/channels in"=w386, "error in"=w387) -> ("task out"=w388:refnum<k21>, "error out"=w389:errorcluster)  [unwired: 12 in]
          n90 = call <vilib>:"DAQmx Clear Task.vi"("task in"=w388, "error in"=w389) -> ("error out"=w383:errorcluster)  [unwired: 13 in]
        }
      }
      n91 = call <vilib>:"DAQmx Create Task.vi"("new task name"="Adiabatic Loading", "auto cleanup"=FALSE, "global virtual channels"=w332, "error in"=w338) -> ("task out"=w354:refnum<k21>, "error out"=w355:errorcluster)  [unwired: 10 in]
      n92 = call-poly <vilib>:"DAQmx Timing.vi"("task/channels in"=w354, "sample mode"=w375, "rate"=w356, "source"=tag "/Dev5/Ctr0InternalOutput", "error in"=w355) -> ("task out"=w359:refnum<k21>, "error out"=w358:errorcluster)  [unwired: 9 in]
      n93 = call-poly <vilib>:"DAQmx Write.vi"("task/channels in"=w359, "data"=w330, "timeout"=10.0, "error in"=w358) -> ("task out"=w360:refnum<k21>, "error out"=w345:errorcluster)  [unwired: 9 in, 1 out]
      n94 = call <vilib>:"DAQmx Create Task.vi"("new task name"="Counter Output", "auto cleanup"=FALSE, "error in"=w345) -> ("task out"=w346:refnum<k21>, "error out"=w344:errorcluster)  [unwired: 11 in]
      n95 = call-poly <vilib>:"DAQmx Create Virtual Channel.vi"("task in"=w346, "frequency"=w356, "counter"=tag "Dev5/ctr0", "error in"=w344, "idle state"=w363) -> ("task out"=w353:refnum<k21>, "error out"=w372:errorcluster)  [unwired: 9 in]
      n96 = call-poly <vilib>:"DAQmx Timing.vi"("task/channels in"=w353, "sample mode"=w371, "samples per channel"=w329, "error in"=w372) -> ("task out"=w367:refnum<k21>, "error out"=w370:errorcluster)  [unwired: 10 in]
      n97 = call-poly <vilib>:"DAQmx Trigger.vi"("task/channels in"=w367, "source"=tag "/Dev5/PFI0", "edge"=w365, "error in"=w370) -> ("task out"=w368:refnum<k21>, "error out"=w369:errorcluster)  [unwired: 10 in]
      n98 = property class="DAQmx Trigger"(reference=w368, error in=w369, "Start:More:Retriggerable"=TRUE ("Start.Retriggerable")) -> (reference out=w366:refnum<k21>, error out=w361:errorcluster)
      n99 = call <vilib>:"DAQmx Start Task.vi"("task/channels in"=w360, "error in"=w361) -> ("task out"=→"6221 adiabatic loading task out":refnum<k21>, "error out"=w362:errorcluster)  [unwired: 12 in]
      n100 = call <vilib>:"DAQmx Start Task.vi"("task/channels in"=w366, "error in"=w362) -> ("task out"=→"6221 counter task out":refnum<k21>, "error out"=w333:errorcluster)  [unwired: 12 in]
      n101 = call <vilib>:"Simple Error Handler.vi"("type of dialog (OK msg:1)"=w374, "error in (no error)"=w333) -> ("error out"=→"error out":errorcluster)  [unwired: 3 in, 4 out]
      "wvfrm size" <- w329
    }
  }
